vi "IV getdata.vi"(0 "pointnr":i32, 5 "x":dbl, 7 "y":dbl, 9 "z":dbl, 11 "error in (no error)":errorcluster) -> (4 "pointnr out":i32, 6 "x out":dbl, 8 "y out":dbl, 10 "z out":dbl, 14 "return type":i32, 15 "error out":errorcluster)   [LabVIEW 2020, in "IVIUM_remdriver.lvlib"]
uses:
  IVIUM_remdriver.lvlib
  SEC Software V4.9/Dependencies/Drivers and Aux files/IVIUM/IVIUM_remdriver.dll
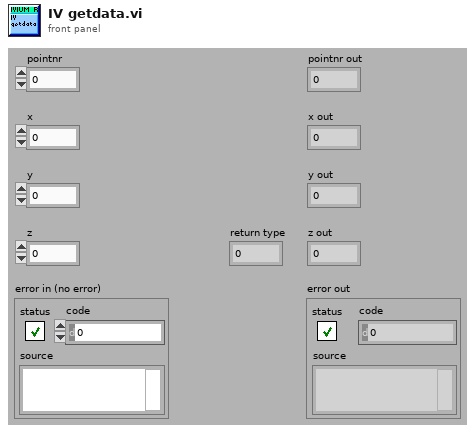
[diagram p1: front panel]
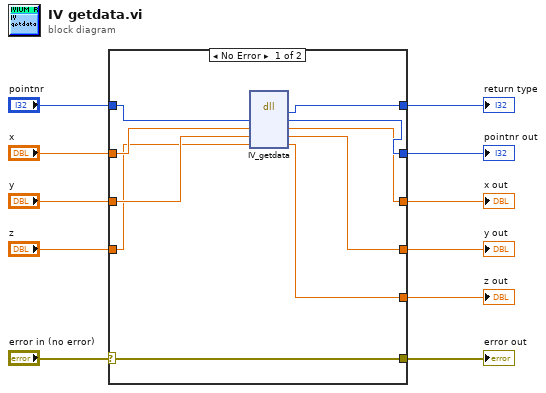
[diagram p0: block diagram]
diagram:
  n1 = case shown="No Error" "error in (no error)" {
    selector: "error in (no error)" -> [w21 w26]
    tunnel: [w21 w26] -> w10
    tunnel: [w20 _] -> w9
    tunnel: "pointnr" -> [w19 w25]
    tunnel: [w18 w25] -> w7
    tunnel: "x" -> [w17 w24]
    tunnel: [w16 w24] -> w5
    tunnel: "y" -> [w15 w23]
    tunnel: [w14 w23] -> w3
    tunnel: "z" -> [w13 w22]
    tunnel: [w12 w22] -> w1
    frame No Error {
      n2 = dll-call lib="C:/Users/Benj/Desktop/SEC Software V4.9/Dependencies/Drivers and Aux files/IVIUM/IVIUM_remdriver.*" fn="IV_getdata"("pointnr"=w19, "x"=w17, "y"=w15, "z"=w13) -> (w20:i32, "pointnr"=w18:i32, "x"=w16:dbl, "y"=w14:dbl, "z"=w12:dbl)  [unwired: 3 in, 2 out]
    }
    frame Error {
    }
  }
  "return type" <- w9
  "pointnr out" <- w7
  "x out" <- w5
  "y out" <- w3
  "z out" <- w1
  "error out" <- w10
